vi "fligh_simulator.vi"() -> ()   [LabVIEW 2017]
uses:
  <vilib>/Utility/miscctls.llb/LV3DPointTypeDef.ctl
  nmea/NMEA_GPVTG-data.ctl
  nmea/NMEA_Mode.ctl
  nmea/NMEA_GPRMC-data.ctl
  nmea/NMEA_LatitudeDirection.ctl
  nmea/NMEA_LongitudeDirection.ctl
  nmea/NMEA_GPGGA-data.ctl
  nmea/NMEA_GPS-Quality.ctl
  Program Files (x86)/National Instruments/LabVIEW 2017/examples/Instrument IO/Serial/support/Serial - Settings.ctl
  Program Files (x86)/National Instruments/LabVIEW 2017/examples/Instrument IO/Serial/support/Serial - XON-XOFF Characters.ctl
  Program Files (x86)/National Instruments/LabVIEW 2017/examples/Instrument IO/Serial/support/Serial - ASCII Characters.ctl
  <vilib>/Instr/_visa.llb/VISA Flush IO Buffer Mask.ctl
  Simflight/Attachments from Google Maps in LabVIEW/Attachments from Google Maps in LabVIEW/Google Maps_LV2012_NI Verified/Google Maps_LV2012_NI Verified/SubVIs/States.ctl
  Program Files (x86)/National Instruments/LabVIEW 2017/examples/Connectivity/Web Services/Weather Monitor/Application/Weather Data.ctl
  <vilib>/Instr/_visa.llb/VISA Configure Serial Port (Instr).vi
  Attitude Indicator 2012 NIVerified/Attitude Indicator 2012 NIVerified/lv-attitudecontrol.lvlib
  Downloads/NMEA_v1.1.2 LV2014/NMEA_v1.1/NMEA.lvlib
  Program Files (x86)/National Instruments/LabVIEW 2017/examples/Connectivity/Web Services/Weather Monitor/Application/Weather Data.lvlib
panel:
  in  "sagsol":dbl(slide) scale=-128.0..128.0
  in  "yukarý":dbl(slide) scale=-128.0..128.0
  out "Waveform Graph":dbl[](graph)
  out "Numeric":dbl format="%#_5g"
  in  "Stop 4":bool
  out "Temperature":dbl
  out "Pressure":dbl
  out "Wind Speed":dbl
  out "Wind Direction":dbl
  in  "Update interval":i32=1000
  in  "Slicon L.":refnum<visa-resource-name>="COM1"
  in  "PROLIFIC":refnum<visa-resource-name>
  out "?":dbl format="%#_4g"
  out "GPS Connection":bool
  in  "WebBrowser":refnum<k7>(container)
  in  "Path Color":u32(colorbox)=16729106
  in  "Weight":i32=7
  in  "Location 1":string(combo)="A"
  in  "Location 2":string(combo)="B"
  in  "Latitude":dbl=51.4062 format="%#.6g"
  in  "Longitude":dbl=-1.3070000000000026 format="%#.6g"
  in  "Zoom":sgl=16.0 format="%#.1g"
  in  "Size Y":dbl=650.0
  in  "Size X":dbl=450.0
  in  "Map Format":string(combo)="roadmap"
  in  "Stop 3":bool
  in  "Add Marker?":bool
  in  "Show Path?":bool
  in  "Refresh Button":bool
  out "Gravity":dbl
  out "Acceleration Y":dbl(slide) scale=-1000.0..1000.0
  out "Acceleration X":dbl(slide) scale=-1000.0..1000.0
  out "ivme z":string
  out "ivme y":string
  out "ivme x":string
  out "Gyro Z":dbl(slide) scale=-1000.0..1000.0
  out "Gyro Y":dbl(slide) scale=-90.0..90.0
  out "Gyro X":dbl(slide) scale=-90.0..90.0
  out "gyro y":string
  out "gyro x":string
  out "Speed in km/h":dbl
  out "PRESSURE\n(ATM)":dbl(knob) scale=0.9..1.2
  out "XY Graph 3":cluster{dbl[], dbl[]}(graph)={[1.6583], [1.60678]}
  out "XY Graph 2":cluster{dbl[], dbl[]}(graph)={[1.6583], [1.60678]}
  out "Battery":dbl(slide) scale=0.1..100.0
  out "Battery":bool
  out "Communication":bool
  out "Temperature":bool
  out "Altitude":bool
  out "Flight Mode":string
  out "Flying":bool
  out "GPS-Quality":T1
  out "Universal\nTime\nCoordinated":timestamp format="%<%I:%M:%S>T"
  out "Altitude":dbl(slide) scale=0.0..500.0
  out "Number of Satellites":i32
  out "Temperature":dbl(slide) scale=0.0..100.0
  out "Speed in Knots":dbl(knob) scale=0.0..10.0
  out "Rx":dbl
  out "Temperature":dbl
  out "Ry":dbl
  out "BASINÇ ATM":dbl
  out "gyro z":string
  out "ry":string
  out "rx":string
  out "BASINÇ":string
  out "Temperature":string
  in  "Termination Character":u8=10 format="%.0x"
  in  "End Write on Termination Character?":bool=TRUE
  in  "XON/XOFF Characters":T2={"XON"=enum."DC1", "XOFF"=enum."DC3"}
  in  "Serial Settings":T4={"baud rate"=9600, "data bits"=8, "parity"=enum."None", "stop bits"=10, "flow control"=0} {"flow control" items=["None"=0, "XON/XOFF"=1, "RTS/CTS"=2, "DTR/DSR"=4]; "stop bits" items=["1.0"=10, "1.5"=15, "2.0"=20]; "data bits" min=5 max=8 step=1; "baud rate" items=["75"=75, "110"=110, "134"=134, "150"=150, "300"=300, "600"=600, "1200"=1200, "1800"=1800, "2400"=2400, "4800"=4800, "7200"=7200, "9600"=9600, "14400"=14400, "19200"=19200, "28800"=28800, "38400"=38400, "56000"=56000, "57600"=57600, "115200"=115200, "128000"=128000, "230400"=230400]}
  in  "End Read on Termination Character?":bool=TRUE
  out "Response":string
  in  "Read Count":u32=1000
  in  "connect":bool
  in  "Stop 2":bool
  in  "Buffer Size":u32=6400
  out "$GPGGA-message_OUT":T5={"TimeStamp"=timestamp(0 s since 1904-01-01), "Latitude"=0.0, "Latitude-Direction"=enum."", "Longitude"=1.0, "Longitude-Direction"=enum."", "GPS-Quality"=enum."GPS fix (SPS)", "Number of Satellites"=0, "Horizontal Dilution of Precision"=0.0, "Altitude above Mean-Sea-Level"=0.0, "Geoidal separation"=0.0, "Time since last DGPS update"=0.0, "DGPS reference station ID"=0} {"Time since last DGPS update" format="%.02f [s]"; "Geoidal separation" format="%.02f [m]"; "Altitude above Mean-Sea-Level" format="%.02f [m]"; "Horizontal Dilution of Precision" format="%.02f [HDOP]"; "Longitude" format="%0.4f [long]"; "Latitude" format="%.04f [lat]"; "TimeStamp" format="%<%.2X>T"}
  out "LATITUDE":dbl
  out "LONGITUDE":dbl
  out "Data":string[][](table)
  out "$GPRMC-message_OUT":T8={"TimeStamp"=timestamp(0 s since 1904-01-01), "Validity"=FALSE, "Latitude"=0.0, "Latitude-Direction"=enum."North", "Longitude"=0.0, "Longitude-Direction"=enum."East", "Speed in knots"=0.0, "True course"=0.0, "Date Stamp"=timestamp(0 s since 1904-01-01), "Magnetic Variation (East/West)"=0.0} {"Magnetic Variation (East/West)" format="%.02f [deg]"; "Date Stamp" format="%<%x>T"; "True course" format="%.02f [deg]"; "Speed in knots" format="%.02f [kts]"; "Longitude" format="%0.4f [long]"; "Latitude" format="%.04f [lat]"; "TimeStamp" format="%<%.2X>T"}
  out "$GPVTG-message_OUT":T9={"True Course over Ground"=0.0, "Magnetic Course over Ground"=0.0, "Speed over Ground in knots"=0.0, "Speed over Ground in km/h"=1.0, "Mode"=""} {"Speed over Ground in km/h" format="%.02f [km/h]"; "Speed over Ground in knots" format="%.02f [kts]"; "Magnetic Course over Ground" format="%.02f [deg]"; "True Course over Ground" format="%.02f [deg]"}
  out "NMEA":string
  in  "Stop":bool
  in  "Control 1":T11 {"X" scale=-90.0..90.0; "Y" scale=-180.0..180.0; "Z" scale=0.0..360.0}
  in  "stop":bool
  in  "pusula":dbl(slide) max=360.0 scale=0.0..360.0
  in  "pusula stop":bool
  out "Gauge":dbl(knob) scale=0.0..360.0
  in  "Attitude Indicator":refnum<vi>(3d-picture)
  # "Flight Status"
  # "UTC"
  # "NOTIFICATIONS"
  # "STATION"
  # "SELCUK ALTINAY\nHAKAN GURBUZ"
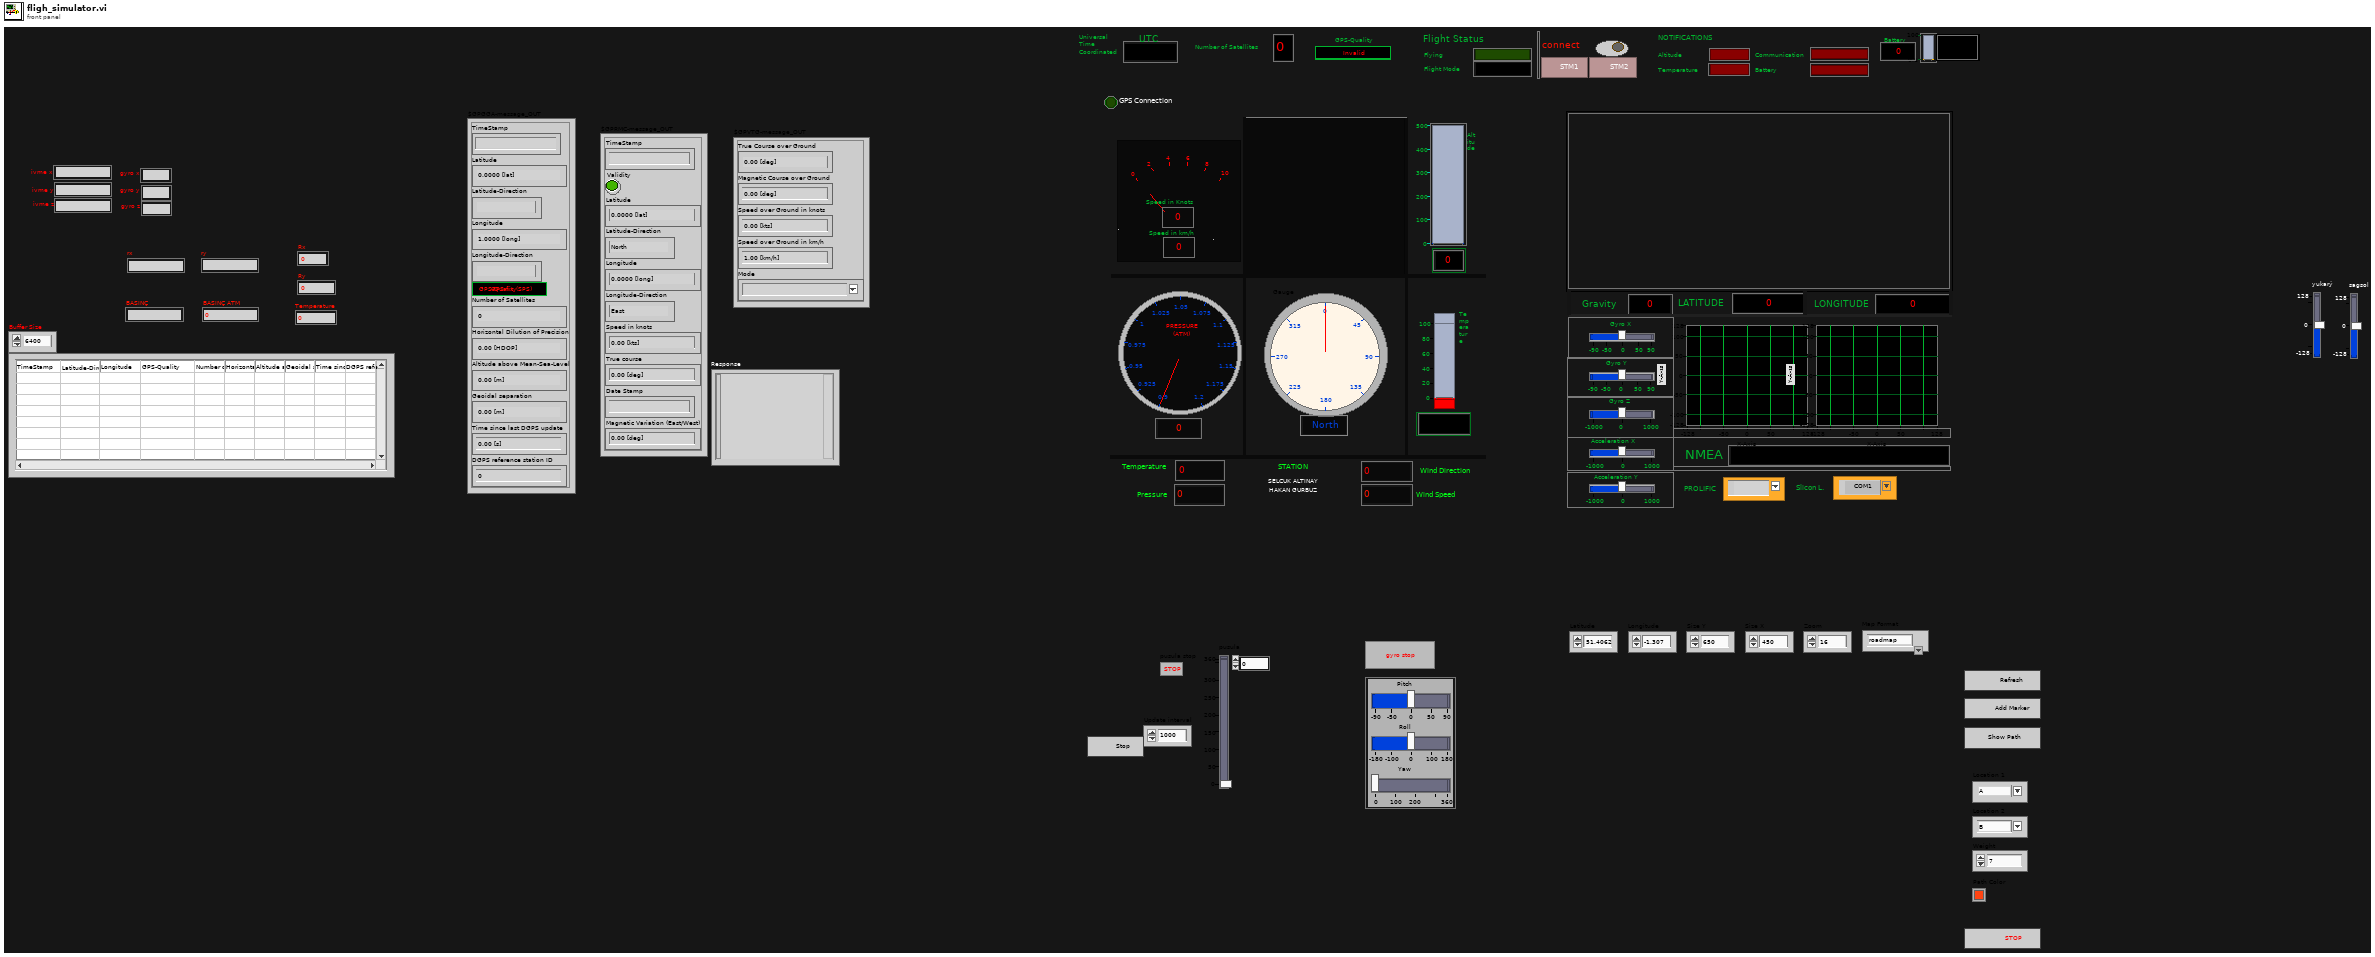
[diagram p1: front panel]
types:
  T1 = typedef "NMEA.lvlib/NMEA_GPS-Quality.ctl" = enum16{"Invalid", "GPS fix (SPS)", "DGPS fix", "PPS fix", "Real Time Kinematic", "Float RTK", "estimated", "Manual input mode", "Simulation mode"}
  T2 = typedef "Serial - XON-XOFF Characters.ctl" = cluster{"XON":T3, "XOFF":T3}
  T3 = typedef "Serial - ASCII Characters.ctl" = enum16{"NUL", "SOH", "STX", "ETX", "EOT", "ENQ", "ACK", "BEL", "BS", "HT", "LF", "VT", "FF", "CR", "SO", "SI", "DLE", "DC1", "DC2", "DC3", "DC4", "NAK", "SYN", "ETB", "CAN", "EM", "SUB", "ESC", "FS", "GS", "RS", "US", "SP", "!", "\"", "#", "$", "%", "&", "'", "(", ")", "*", "+", ",", "- (-)", ".", "/", "0", "1", "2", "3", "4", "5", "6", "7", "8", "9", ":", ";", "<", "=", ">", "?", "@", "A", "B", "C", "D", "E", "F", "G", "H", "I", "J", "K", "L", "M", "N", "O", "P", "Q", "R", "S", "T", "U", "V", "W", "X", "Y", "Z", "[", "\\", "]", "^", "_", "`", "a", "b", "c", "d", "e", "f", "g", "h", "i", "j", "k", "l", "m", "n", "o", "p", "q", "r", "s", "t", "u", "v", "w", "x", "y", "z", "{", "|", "}", "~"}
  T4 = typedef "Serial - Settings.ctl" = cluster{"baud rate":u32, "data bits":u16, "parity":enum16{"None", "Odd", "Even", "Mark", "Space"}, "stop bits":u16, "flow control":u16}
  T5 = typedef "NMEA.lvlib/NMEA_GPGGA-data.ctl" = cluster{"TimeStamp":timestamp, "Latitude":dbl, "Latitude-Direction":T6, "Longitude":dbl, "Longitude-Direction":T7, "GPS-Quality":T1, "Number of Satellites":i32, "Horizontal Dilution of Precision":dbl, "Altitude above Mean-Sea-Level":dbl, "Geoidal separation":dbl, "Time since last DGPS update":dbl, "DGPS reference station ID":i32}
  T6 = typedef "NMEA.lvlib/NMEA_LatitudeDirection.ctl" = enum16{"", "North", "South"}
  T7 = typedef "NMEA.lvlib/NMEA_LongitudeDirection.ctl" = enum16{"", "East", "West"}
  T8 = typedef "NMEA.lvlib/NMEA_GPRMC-data.ctl" = cluster{"TimeStamp":timestamp, "Validity":bool, "Latitude":dbl, "Latitude-Direction":T6, "Longitude":dbl, "Longitude-Direction":T7, "Speed in knots":dbl, "True course":dbl, "Date Stamp":timestamp, "Magnetic Variation (East/West)":dbl}
  T9 = typedef "NMEA.lvlib/NMEA_GPVTG-data.ctl" = cluster{"True Course over Ground":dbl, "Magnetic Course over Ground":dbl, "Speed over Ground in knots":dbl, "Speed over Ground in km/h":dbl, "Mode":T10}
  T10 = typedef "NMEA.lvlib/NMEA_Mode.ctl" = string
  T11 = typedef "LV3DPointTypeDef.ctl" = cluster{"X":sgl, "Y":sgl, "Z":sgl}
  T12 = cluster{"Marker":string, "Path":string, "Markers Coordinates":string[][]}
  T13 = typedef "States.ctl" = enum16{"Wait on Event", "Update Map", "Add Marker", "Show Path", "Shutdown"}
  T14 = typedef "VISA Flush IO Buffer Mask.ctl" = u16
  T15 = typedef "Weather Data.lvlib/Weather Data.ctl" = cluster{"Temperature":dbl, "Pressure":dbl, "Wind Speed":dbl, "Wind Direction":dbl}
  T16 = typedef "lv-attitudecontrol.lvlib/AttitudeHandle.ctl" = cluster{"First Scene Object":refnum<vi>, "Drum":refnum<vi>, "Window":refnum<vi>, "Dial":refnum<vi>, "Scene Graph":refnum<vi>, "Last Drum Pitch":dbl, "Last Drum Roll ":dbl, "Last Dial Roll":dbl}
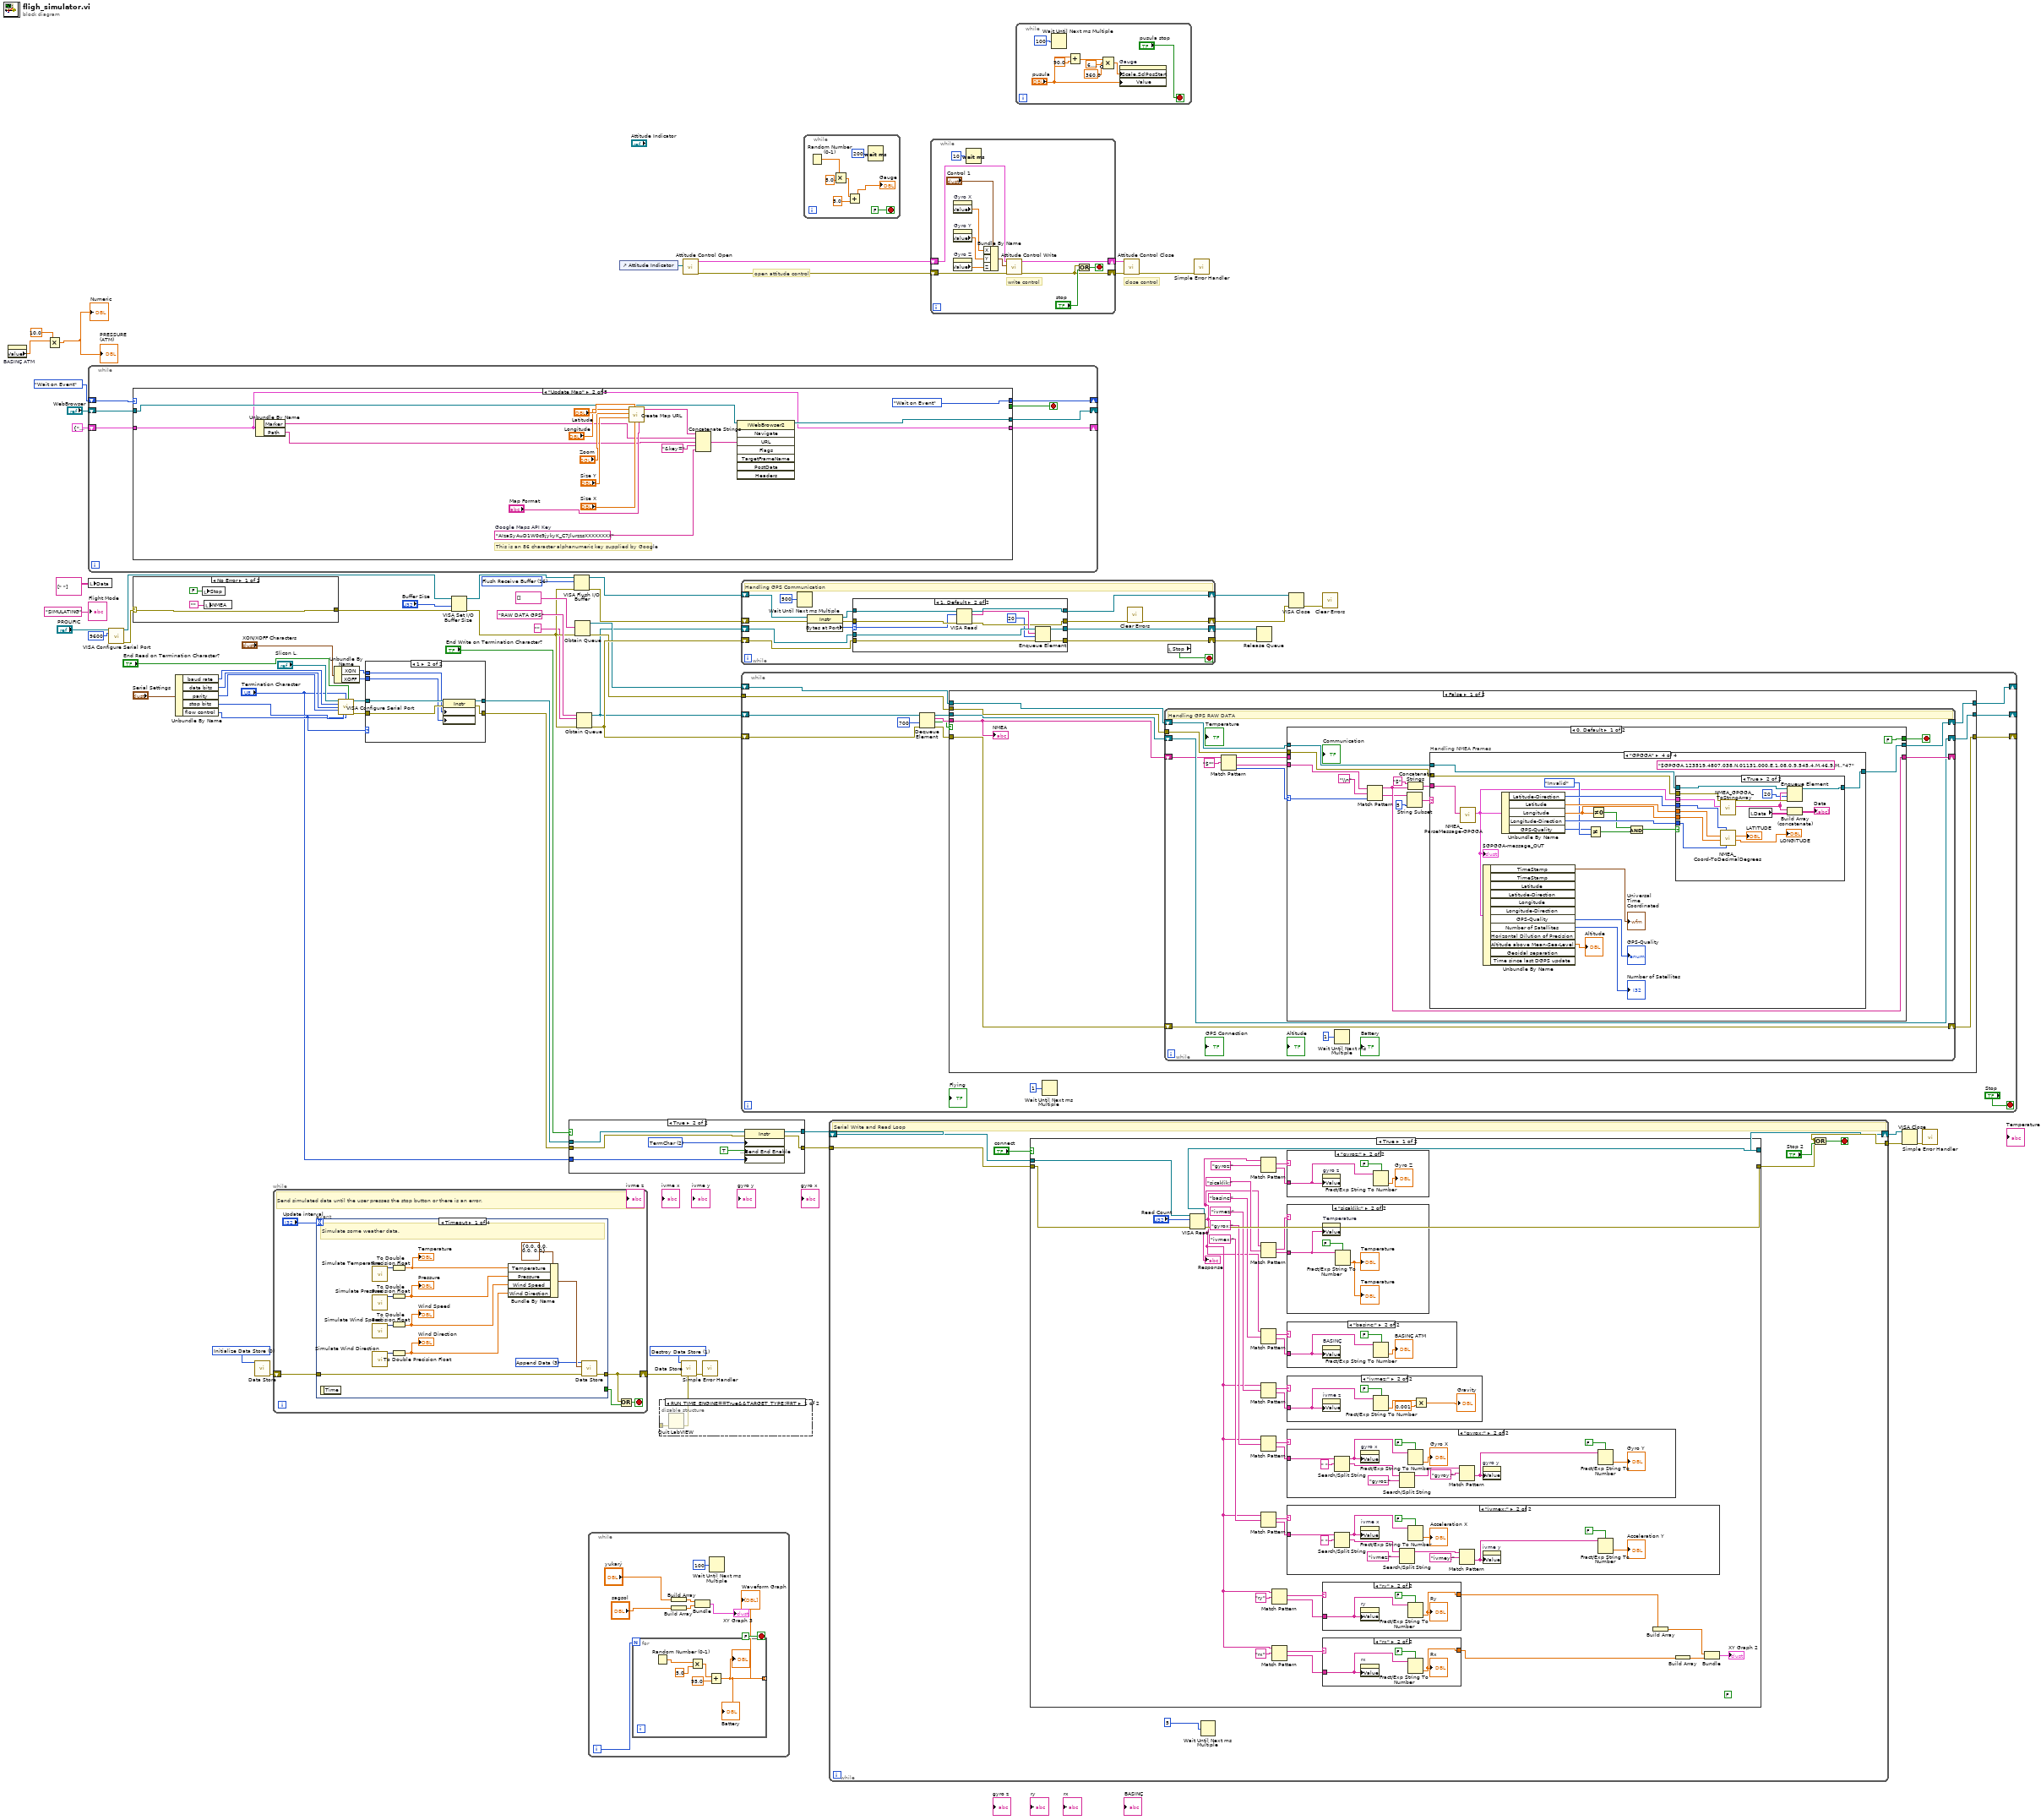
[diagram p0: block diagram]
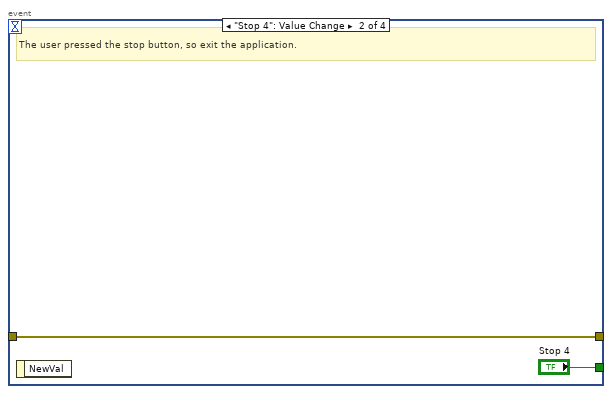
[diagram p3: hidden frame]
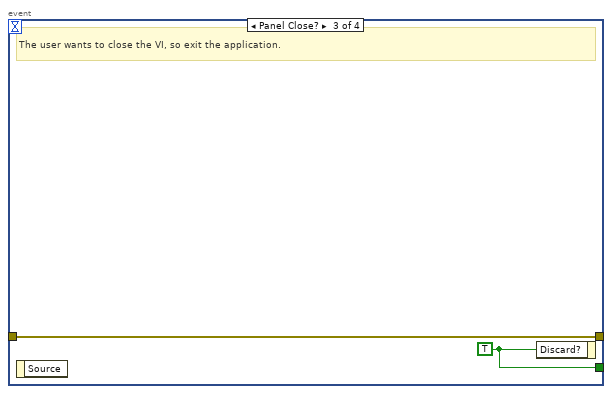
[diagram p4: hidden frame]
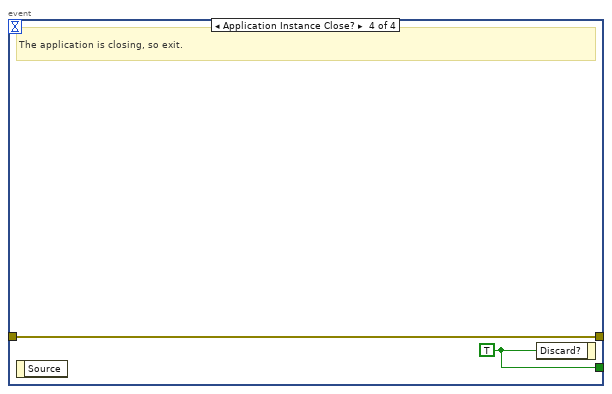
[diagram p5: hidden frame]
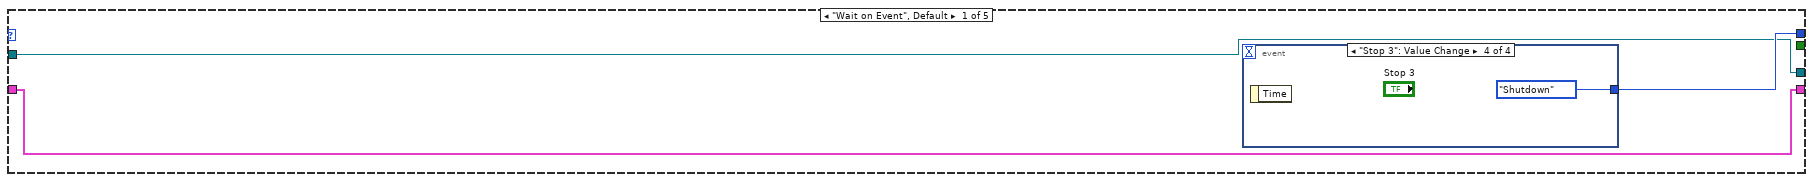
[diagram p6: hidden frame]
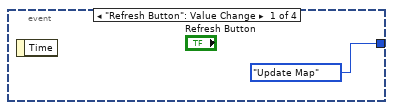
[diagram p7: hidden frame]
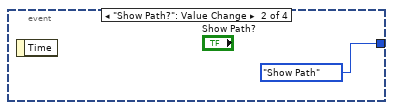
[diagram p8: hidden frame]
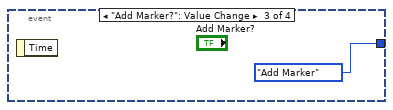
[diagram p9: hidden frame]
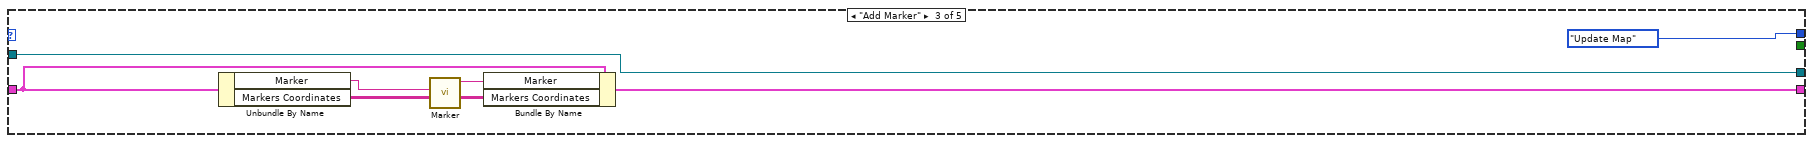
[diagram p10: hidden frame]
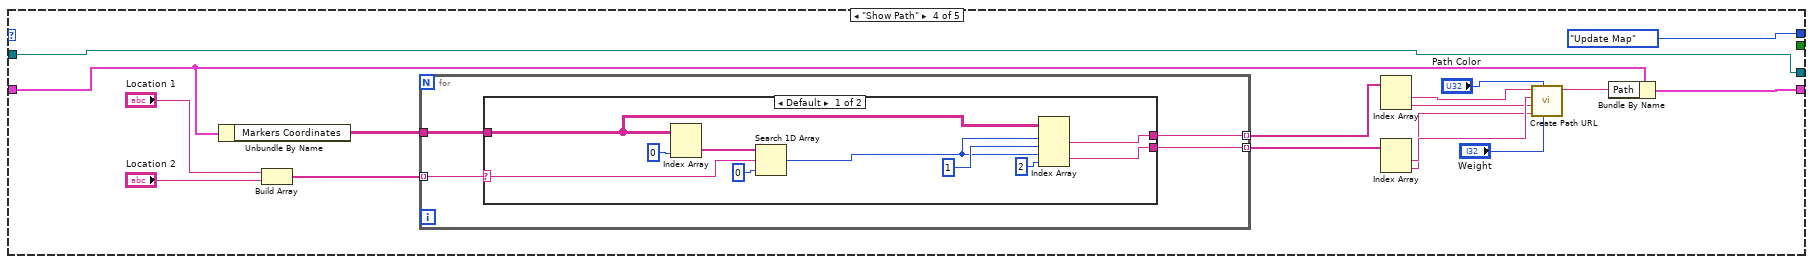
[diagram p11: hidden frame]
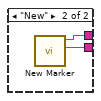
[diagram p12: hidden frame]
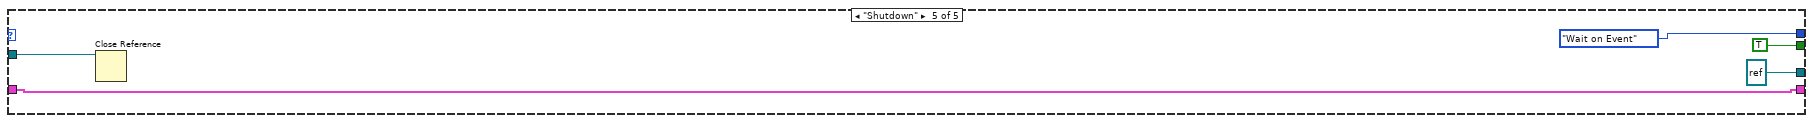
[diagram p13: hidden frame]
diagram:
  w8 = u16 1 items=["Initialize Data Store", "Destroy Data Store", "Clear Data", "Append Data", "Get Last Data", "Get All Data"] ("action")
  w5 = u16 0 items=["Initialize Data Store", "Destroy Data Store", "Clear Data", "Append Data", "Get Last Data", "Get All Data"] ("action")
  w49 = T14 16 items=["Flush Receive Buffer"=16, "Write Transmit Buffer to Device"=32, "Flush Receive Buffer (No I/O)"=64, "Flush Transmit Buffer"=128] ("Mask")
  # "close control"
  # "open attitude control"
  n1 = property on="BASINÇ ATM" class="DigNum (strict)"() -> ("Value"=w3:dbl)  [unwired: 2 in, 2 out]
  n2 = Multiply(x=w3, y=10.0) -> (x*y=→"PRESSURE\n(ATM)" →"Numeric":dbl)
  n3 = while {
    shift-right: [w72] -> _
    shift-left: States."Wait on Event" -> [w71]
    shift-right: [w69] -> _
    shift-left: "WebBrowser" -> [w68]
    shift-right: [w66] -> _
    shift-left: T12 {"Marker"="", "Path"="", "Markers Coordinates"=[]} -> [w67]
    stop <- w70 stop-if-true
    n4 = case shown="\"Update Map\"" w71 {
      tunnel: [w75 States."Wait on Event" States."Update Map" States."Update Map" States."Wait on Event"] -> w72
      tunnel: [_ _ _ _ TRUE] -> w70
      tunnel: w68 -> [w74 w87 w103 w120 w140]
      tunnel: [w74 w86 w103 w120 refnum<k7> refnum ("WebBrowser")] -> w69
      tunnel: w67 -> [w73 w80 w99 w109 w137]
      tunnel: [w73 w80 w96 w108 w137] -> w66
      frame "Wait on Event", Default {
        n5 = event shown="[3] \"Stop 3\": Value Change" {
          selector: _ -> [_ _ _ _]
          dyn-events: _ -> [_ _ _ _]
          timeout: _ -> [_ _ _ _]
          tunnel: [States."Update Map" States."Show Path" States."Add Marker" States."Shutdown"] -> w75
          event "Refresh Button": Value Change {
            n6 = event-data() -> ()  [unwired: 1 in, 1 out]
          }
          event "Show Path?": Value Change {
            n7 = event-data() -> ()  [unwired: 1 in, 1 out]
          }
          event "Add Marker?": Value Change {
            n8 = event-data() -> ()  [unwired: 1 in, 1 out]
          }
          event "Stop 3": Value Change {
            n9 = event-data() -> ()  [unwired: 1 in, 1 out]
          }
        }
      }
      frame "Update Map" {
        w83 = "AIzaSyAuD1W0c9jykyK_C7JlurzzsXXXXXXXX"  # Google Maps API Key
        # "This is an 86 character alphanumeric key supplied by Google"
        n10 = Unbundle By Name(w80) -> ("Marker"=w82:string, "Path"=w81:string)
        n11 = call "Create Map URL.vi"("Map Format"="Map Format", "X"="Size X", "Lat"="Latitude", "Y"="Size Y", "Zoom"="Zoom", "Lon"="Longitude") -> ("String"=w89:string)  [unwired: 5 in]
        n12 = Concatenate Strings(w89, w82, w81, "&key=" ("string"), w83) -> (w88:string)
        n13 = invoke class="IWebBrowser2" method="Navigate"(reference=w87, "URL"=w88) -> (reference out=w86:refnum<k7>)  [unwired: 6 in, 7 out]
      }
      frame "Add Marker" {
        n14 = Unbundle By Name(w99) -> ("Marker"=w101:string, "Markers Coordinates"=w100:string[][])
        n15 = call "Marker.vi"("Markers in"=w100, "Initial String"=w101) -> ("Markers out"=w97:string[][], "Balloon"=w98:string)  [unwired: 8 in]
        n16 = Bundle By Name(cluster=w99, "Marker"=w98, "Markers Coordinates"=w97) -> (w96:T12)
      }
      frame "Show Path" {
        n17 = Unbundle By Name(w109) -> ("Markers Coordinates"=w111:string[][])
        n18 = Build Array("Location 1", "Location 2") -> (w116:string[])
        n19 = for {
          tunnel: w116 -> [w124] mode=indexing
          tunnel: [w123] -> w115 mode=indexing
          tunnel: [w122] -> w114 mode=indexing
          tunnel: w111 -> [w121]
          n20 = case shown="Default" w124 {
            selector: w124 -> [w125 _]
            tunnel: [w127 w136] -> w123
            tunnel: [w126 w135] -> w122
            tunnel: w121 -> [w128 _]
            frame Default {
              n21 = Index Array(array=w128, index (col)=0 ("disabled index (col)")) -> (element=w129:string[])  [unwired: 1 in]
              n22 = Search 1D Array(1D array=w129, element=w125, start index (0)=0) -> (index of element=w132:i32)
              n23 = Index Array(array=w128, index (row) #1=w132, index (col) #1=1 ("disabled index (col)"), index (row) #2=w132, index (col) #2=2 ("disabled index (col)")) -> (element #1=w127:string, element #2=w126:string)
            }
            frame "New" {
              n24 = call "New Marker.vi"() -> ("Longitude"=w135:string, "Latitude"=w136:string)  [unwired: 10 in]
            }
          }
        }
        n25 = Index Array(array=w115) -> (element #1=w112:string, element #2=w105:string)  [unwired: 2 in]
        n26 = Index Array(array=w114) -> (element #1=w106:string, element #2=w104:string)  [unwired: 2 in]
        n27 = call "Create Path URL.vi"("Weight"="Weight", "Path Collor"="Path Color", "Long Point 2"=w104, "Lat Point 2"=w105, "Long Point 1"=w106, "Lat Point 1"=w112) -> ("String 4"=w110:string)  [unwired: 5 in]
        n28 = Bundle By Name(cluster=w109, "Path"=w110) -> (w108:T12)
      }
      frame "Shutdown" {
        n29 = Close Reference(reference=w140) -> ()  [unwired: 1 in, 1 out]
      }
    }
  }
  n30 = local write "Data"(string[][] [[" "]]) -> ()
  n31 = call-poly "VISA Configure Serial Port"("VISA resource name"="PROLIFIC", "baud rate (9600)"=u32 9600) -> ("VISA resource name out"=w50:refnum<visa-resource-name>, "error out"=w41:errorcluster)  [unwired: 12 in]
  n32 = case shown="No Error" w41 {
    selector: w41 -> [w143 w145]
    tunnel: [w143 w145] -> w39
    frame No Error {
      n33 = local write "Stop"(FALSE ("STOP")) -> ()
      n34 = local write "NMEA"("") -> ()
    }
    frame Error {
    }
  }
  n35 = Unbundle By Name("Serial Settings") -> ("baud rate"=w28:u32, "data bits"=w29:u16, "parity"=w30:enum16{"None", "Odd", "Even", "Mark", "Space"}, "stop bits"=w31:u16, "flow control"=w22:u16)
  n36 = call "Data Store.vi"("action"=w5) -> ("error out"=w6:errorcluster)  [unwired: 9 in, 1 out]
  n37 = while {
    shift-right: [w148] -> w7
    shift-left: w6 -> [w150]
    stop <- w149 stop-if-true
    # "Send simulated data until the user presses the stop button or there is an error."
    n38 = event shown="[0] Timeout" {
      selector: _ -> [_ _ _ _]
      dyn-events: _ -> [_ _ _ _]
      timeout: "Update interval" -> [_ _ _ _]
      tunnel: w150 -> [w159 w165 w167 w169]
      tunnel: [w157 w165 w167 w169] -> w148
      tunnel: [_ "Stop 4" w166 w168] -> w146
      event Timeout {
        w151 = u16 3 items=["Initialize Data Store", "Destroy Data Store", "Clear Data", "Append Data", "Get Last Data", "Get All Data"] ("action")
        # "Simulate some weather data."
        n39 = event-data() -> ()  [unwired: 1 in, 1 out]
        n40 = call "Simulate Temperature"() -> ("DC with Uniform Noise"=w156:dynamicdata)  [unwired: 5 in, 10 out]
        n41 = call "Simulate Pressure"() -> ("Sine with Uniform Noise"=w162:dynamicdata)  [unwired: 8 in, 7 out]
        n42 = call "Simulate Wind Speed"() -> ("Sine with Uniform Noise"=w161:dynamicdata)  [unwired: 8 in, 7 out]
        n43 = call "Simulate Wind Direction"() -> ("Sine with Uniform Noise"=w160:dynamicdata)  [unwired: 8 in, 7 out]
        n44 = To Double Precision Float(number=w156) -> (double precision float=w155:dbl)
        "Temperature" <- w155
        n45 = To Double Precision Float(number=w162) -> (double precision float=w154:dbl)
        "Pressure" <- w154
        n46 = To Double Precision Float(number=w161) -> (double precision float=w153:dbl)
        "Wind Speed" <- w153
        n47 = To Double Precision Float(number=w160) -> (double precision float=w152:dbl)
        "Wind Direction" <- w152
        n48 = Bundle By Name(cluster=T15 {"Temperature"=0.0, "Pressure"=0.0, "Wind Speed"=0.0, "Wind Direction"=0.0} ("Weather Data"), "Temperature"=w155, "Pressure"=w154, "Wind Speed"=w153, "Wind Direction"=w152) -> (w158:T15)
        n49 = call "Data Store.vi"("error in (no error)"=w159, "new weather data"=w158, "action"=w151) -> ("error out"=w157:errorcluster)  [unwired: 7 in, 1 out]
      }
      event "Stop 4": Value Change {
        # "The user pressed the stop button, so exit the application."
        n50 = event-data() -> ()  [unwired: 1 in, 1 out]
      }
      event Panel Close? {
        w166 = TRUE ("Discard?")
        # "The user wants to close the VI, so exit the application."
        n51 = event-data() -> ()  [unwired: 1 in, 1 out]
        n52 = event-data("Discard?"=w166) -> ()  [unwired: 1 in, 1 out]
      }
      event Application Instance Close? {
        w168 = TRUE ("Discard?")
        # "The application is closing, so exit."
        n53 = event-data() -> ()  [unwired: 1 in, 1 out]
        n54 = event-data("Discard?"=w168) -> ()  [unwired: 1 in, 1 out]
      }
    }
    n55 = Or(x=w148, y=w146) -> (x .or. y?=w149:bool)
  }
  n56 = Unbundle By Name("XON/XOFF Characters") -> ("XON"=w21:T3, "XOFF"=w20:T3)
  n57 = call-poly "VISA Configure Serial Port"("VISA resource name"="Slicon L.", "termination char\n(0xA = '\\n' = LF)"="Termination Character", "Enable Termination\nChar (T)"="End Read on Termination Character?", "baud rate (9600)"=w28, "data bits (8)"=w29, "parity (0:none)"=w30, "stop bits (10: 1 bit)"=w31, "flow control (0:none)"=w22) -> ("VISA resource name out"=w32:refnum<visa-resource-name>, "error out"=w33:errorcluster)  [unwired: 2 in, 4 out]
  n58 = case shown="1" w22 {
    tunnel: [w170 w177] -> w19
    tunnel: [w171 w176] -> w17
    tunnel: w33 -> [w170 w175]
    tunnel: w32 -> [w171 w174]
    tunnel: w21 -> [_ w173]
    tunnel: w20 -> [_ w172]
    frame Default {
    }
    frame 1 {
      n59 = property class="Instr"(reference=w174, error in=w175, "Serial Settings:Flow Control XON Character"=w173, "Serial Settings:Flow Control XOFF Character"=w172) -> (reference out=w176:refnum<visa-resource-name>, error out=w177:errorcluster)
    }
  }
  n60 = VISA Set I/O Buffer Size(VISA resource name=w50, size (4096)="Buffer Size", error in (no error)=w39) -> (VISA resource name out=w59:refnum<visa-resource-name>, error out=w38:errorcluster)  [unwired: 1 in]
  n61 = case shown="True" "End Write on Termination Character?" {
    tunnel: w17 -> [w178 w186]
    tunnel: w19 -> [w179 w185]
    tunnel: [w178 w184] -> w16
    tunnel: [w179 w183] -> w18
    tunnel: "Termination Character" -> [_ w181]
    frame False {
    }
    frame True {
      w182 = u16 2 items=["None", "LastBit", "TermChar", "Break"] ("Serial Settings:Serial End Mode for Writes")
      n62 = property class="Instr"(reference=w186, error in=w185, "Serial Settings:End Mode for Writes"=w182, "Message Based Settings:Send End Enable"=TRUE, "Message Based Settings:Termination Character"=w181) -> (reference out=w184:refnum<visa-resource-name>, error out=w183:errorcluster)
    }
  }
  n63 = VISA Flush I/O Buffer(VISA resource name=w59, mask (16)=w49, error in (no error)=w38) -> (VISA resource name out=w58:refnum<visa-resource-name>, error out=w57:errorcluster)
  n64 = Obtain Queue(element data type=string[] [], error in (no error)=w38) -> (queue out=w55:refnum<queue>, error out=w54:errorcluster)  [unwired: 3 in, 1 out]
  n65 = Obtain Queue(name (unnamed)="RAW DATA GPS" ("nom (aucun)"), element data type="" ("expression régulière"), error in (no error)=w38) -> (queue out=w45:refnum<queue>, error out=w56:errorcluster)  [unwired: 2 in, 1 out]
  n66 = while {
    i -> [w187]
    stop <- FALSE stop-if-true
    n67 = for {
      N: w187 -> [_]
      tunnel: [w196] -> w188 mode=indexing
      n68 = Random Number (0-1)() -> (number: 0 to 1=w200:dbl)
      n69 = Multiply(x=w200, y=5.0) -> (x*y=w198:dbl)
      n70 = Add(x=w198, y=95.0) -> (x+y=w196:dbl)
      "Battery" <- w196
      "?" <- w196
    }
    "Waveform Graph" <- w188
    n71 = Build Array("yukarý") -> (w195:dbl[])
    n72 = Build Array("sagsol") -> (w194:dbl[])
    n73 = Bundle(w195, w194) -> (→"XY Graph 3":cluster{dbl[], dbl[]})  [unwired: 1 in]
    n74 = Wait Until Next ms Multiple(millisecond multiple=u32 100) -> ()  [unwired: 1 out]
  }
  n75 = control-ref of="Attitude Indicator"() -> (w62:refnum<vi>)
  n76 = call "Data Store.vi"("error in (no error)"=w7, "action"=w8) -> ("error out"=w4:errorcluster)  [unwired: 8 in, 1 out]
  n77 = call "Attitude Control Open.vi"("Scene Graph"=w62) -> ("error out"=w61:errorcluster, "Attitude Control Handle"=w60:T16)  [unwired: 9 in]
  n78 = call <vilib>:"Simple Error Handler.vi"("error in (no error)"=w4) -> ("error out"=w9:errorcluster)  [unwired: 4 in, 4 out]
  n79 = disable-structure shown="RUN_TIME_ENGINE==True&&TARGET_TYPE!=RT" {
    disable-tunnel: w9 -> [_ _]
    frame condition #0 {
      n80 = Quit LabVIEW() -> ()  [unwired: 1 in]
    }
    frame condition #1 (active) {
    }
  }
  n81 = while {
    shift-right: [w211] -> w47
    shift-left: w56 -> [w213]
    shift-right: [w210] -> w44
    shift-left: w58 -> [w209]
    shift-right: [w212] -> w46
    shift-left: w45 -> [w214]
    shift-right: [w202] -> w43
    shift-left: w57 -> [w206]
    stop <- w201 stop-if-true
    # "Handling GPS Communication"
    n82 = Wait Until Next ms Multiple(millisecond multiple=u32 500 ("attente (ms)")) -> ()  [unwired: 1 out]
    n83 = property class="Instr"(reference=w209, error in=w206) -> (reference out=w208:refnum<visa-resource-name>, error out=w205:errorcluster, "Bytes at Port"=w203:u32)
    n84 = case shown="1, Default" w203 {
      selector: w203 -> [_ w220]
      tunnel: w214 -> [w215 w229]
      tunnel: w213 -> [w216 w228]
      tunnel: [w215 w227] -> w212
      tunnel: [w216 w226] -> w211
      tunnel: [w217 w224] -> w210
      tunnel: w208 -> [w217 w223]
      tunnel: w205 -> [w218 w222]
      tunnel: [w218 w221] -> w204
      frame 0 {
      }
      frame 1, Default {
        n85 = VISA Read(VISA resource name=w223, byte count=w220, error in (no error)=w222) -> (VISA resource name out=w224:refnum<visa-resource-name>, read buffer=w225:string, error out=w221:errorcluster)  [unwired: 1 out]
        n86 = Enqueue Element(queue=w229, element=w225, timeout in ms (-1)=20 ("timeout en ms (-1)"), error in (no error)=w228) -> (queue out=w227:refnum<queue>, error out=w226:errorcluster)  [unwired: 1 out]
      }
    }
    n87 = call <vilib>:"Clear Errors.vi"("error in (no error)"=w204) -> ("error out"=w202:errorcluster)  [unwired: 5 in, 1 out]
    n88 = local read "Stop"() -> (w201:bool)
  }
  n89 = while {
    tunnel: w54 -> [w239]
    shift-right: [w237] -> _
    shift-left: w45 -> [w238]
    shift-right: [w233] -> _
    shift-left: w55 -> [w240]
    shift-right: [w232] -> _
    shift-left: w56 -> [w243]
    stop <- "Stop" stop-if-true
    n90 = Dequeue Element(queue=w238, timeout in ms (-1)=700 ("timeout en ms (-1)"), error in (no error)=w243) -> (queue out=w236:refnum<queue>, element=w242:string, timed out?=w234:bool, error out=w231:errorcluster)
    n91 = case shown="False" w234 {
      tunnel: w242 -> [w244 _]
      tunnel: w240 -> [w251 w324]
      tunnel: w239 -> [w250 _]
      tunnel: [w249 w325] -> w237
      tunnel: w236 -> [w248 w325]
      tunnel: [w247 w324] -> w233
      tunnel: [w246 w323] -> w232
      tunnel: w231 -> [w245 w323]
      frame False {
        n92 = while {
          shift-right: [w262] -> _
          shift-left: w244 -> [w253]
          tunnel: w250 -> [w258]
          shift-right: [w257] -> w249
          shift-left: w248 -> [w257]
          shift-right: [w255] -> w247
          shift-left: w251 -> [w259]
          shift-right: [w254] -> w246
          shift-left: w245 -> [w254]
          stop <- w256 stop-if-true
          # "Handling GPS RAW DATA"
          n93 = Match Pattern(string=w253, regular expression="$*" ("expression régulière")) -> (before substring=w252:string, after substring=w261:string, offset past match=w263:i32)  [unwired: 1 in, 1 out]
          n94 = case shown="0, Default" w263 {
            selector: w263 -> [w274 _]
            tunnel: [w273 w320] -> w262
            tunnel: w261 -> [w275 _]
            tunnel: [FALSE TRUE] -> w256
            tunnel: w259 -> [w268 w321]
            tunnel: w258 -> [w267 _]
            tunnel: [w265 w321] -> w255
            tunnel: w252 -> [_ w320]
            frame 0, Default {
              n95 = Match Pattern(string=w275, regular expression="\\n" ("expression régulière"), offset (0)=w274) -> (before substring=w272:string, after substring=w273:string)  [unwired: 2 out]
              n96 = String Subset(string=w272, length (rest)=5 ("longueur (reste)")) -> (substring=w276:string)  [unwired: 1 in]
              n97 = Concatenate Strings("$" ("expression régulière"), w272) -> (w270:string)
              n98 = case "Handling NMEA Frames" shown="\"GPGGA\"" w276 {
                tunnel: w270 -> [_ w282 w286 w304]
                tunnel: w268 -> [w278 w281 w285 w300]
                tunnel: w267 -> [_ _ _ w299]
                tunnel: [w278 w281 w285 w298] -> w265
                frame " ", Default {
                }
                frame "GPVTG" {
                  (unwired) "$GPVTG,054.7,T,034.4,M,005.5,N,010.2,K*48" ("$GPVTG-message_IN")
                  n99 = call "NMEA_ParseMessage-GPVTG.vi"("$GPVTG-message_IN"=w282) -> ("$GPVTG-message_OUT"=w280:T9)  [unwired: 9 in, 1 out]
                  "$GPVTG-message_OUT" <- w280
                  n100 = Unbundle By Name(w280) -> ("Speed over Ground in km/h"=→"Speed in km/h":dbl)  [unwired: 3 out]
                }
                frame "GPRMC" {
                  (unwired) "$GPRMC,225446,A,4916.45,N,12311.12,W,000.5,054.7,191194,020.3,E*68" ("$GPRMC-message_IN")
                  n101 = call "NMEA_ParseMessage-GPRMC.vi"("$GPRMC-message_IN"=w286) -> ("$GPRMC-message_OUT"=w283:T8)  [unwired: 9 in, 1 out]
                  "$GPRMC-message_OUT" <- w283
                  n102 = Unbundle By Name(w283) -> ("Speed in knots"=→"Speed in Knots":dbl)  [unwired: 11 out]
                }
                frame "GPGGA" {
                  (unwired) "$GPGGA,123519,4807.038,N,01131.000,E,1,08,0.9,545.4,M,46.9,M,,*47" ("data out")
                  n103 = call "NMEA_ParseMessage-GPGGA.vi"("$GPGGA-message_IN"=w304) -> ("$GPGGA-message_OUT"=w290:T5)  [unwired: 9 in, 1 out]
                  "$GPGGA-message_OUT" <- w290
                  n104 = Unbundle By Name(w290) -> ("TimeStamp"=→"Universal\nTime\nCoordinated":timestamp, "GPS-Quality"=→"GPS-Quality":T1, "Number of Satellites"=→"Number of Satellites":i32, "Altitude above Mean-Sea-Level"=→"Altitude":dbl)  [unwired: 8 out]
                  n105 = Unbundle By Name(w290) -> ("Latitude-Direction"=w301:T6, "Latitude"=w302:dbl, "Longitude"=w297:dbl, "Longitude-Direction"=w303:T7, "GPS-Quality"=w292:T1)
                  n106 = Not Equal?(x=w292, y=NMEA_GPS-Quality."Invalid" ("GPS-Quality")) -> (x != y?=w293:bool)
                  n107 = Not Equal To 0?(x=w297) -> (x != 0?=w295:bool)
                  n108 = Compound Arithmetic op=AND(w295, w293) -> (w296:bool)
                  n109 = case shown="True" w296 {
                    tunnel: w303 -> [_ w317]
                    tunnel: w302 -> [_ w307]
                    tunnel: w301 -> [_ w306]
                    tunnel: w290 -> [_ w316]
                    tunnel: w300 -> [w305 w315]
                    tunnel: w299 -> [_ w314]
                    tunnel: [w305 w310] -> w298
                    tunnel: w297 -> [_ w308]
                    frame False {
                    }
                    frame True {
                      n110 = call "NMEA_GPGGA_ToStringArray.vi"("$GPGGA-message_IN"=w316) -> ("$GPGGA-message_OUT"=w312:string[])  [unwired: 9 in, 1 out]
                      n111 = call "NMEA_Coord-ToDecimalDegrees.vi"("Longitude-Direction"=w317, "Latitude-Direction"=w306, "Longitude"=w308, "Latitude"=w307) -> ("Longitude"=→"LONGITUDE":dbl, "Latitude"=→"LATITUDE":dbl)  [unwired: 6 in]
                      n112 = local read "Data"() -> (w311:string[][])
                      n113 = Enqueue Element(queue=w315, element=w312, timeout in ms (-1)=20 ("timeout en ms (-1)"), error in (no error)=w314) -> (queue out=w310:refnum<queue>)  [unwired: 2 out]
                      n114 = Build Array (concatenate)(w312, w311) -> (→"Data":string[][])
                    }
                  }
                }
              }
            }
            frame -1 {
            }
          }
          n115 = Wait Until Next ms Multiple(millisecond multiple=u32 1 ("n millisecondes")) -> ()  [unwired: 1 out]
        }
        "NMEA" <- w244
      }
      frame True {
      }
    }
    n116 = Wait Until Next ms Multiple(millisecond multiple=u32 1 ("n millisecondes")) -> ()  [unwired: 1 out]
  }
  n117 = while {
    stop <- FALSE stop-if-true
    n118 = Random Number (0-1)() -> (number: 0 to 1=w331:dbl)
    n119 = Multiply(x=w331, y=5.0) -> (x*y=w332:dbl)
    n120 = Add(x=w332, y=5.0) -> (x+y=→"Gauge":dbl)
    n121 = Wait (ms)(milliseconds to wait=u32 200) -> ()  [unwired: 1 out]
  }
  n122 = while {
    shift-right: [w333] -> w23
    shift-left: w16 -> [w337]
    tunnel: w18 -> [w336]
    tunnel: [w334] -> w24
    stop <- w339 stop-if-true
    # "Serial Write and Read Loop"
    n123 = case shown="True" "connect" {
      tunnel: [w375 w421] -> w333
      tunnel: w337 -> [w347 w421]
      tunnel: [w373 w420] -> w334
      tunnel: w336 -> [w346 w420]
      frame True {
        (unwired) FALSE
        n124 = VISA Read(VISA resource name=w347, byte count="Read Count", error in (no error)=w346) -> (VISA resource name out=w375:refnum<visa-resource-name>, read buffer=w348:string, error out=w373:errorcluster)  [unwired: 1 out]
        "Response" <- w348
        n125 = Match Pattern(string=w348, regular expression="gyroz:") -> (match substring=w360:string, after substring=w359:string)  [unwired: 1 in, 2 out]
        n126 = Match Pattern(string=w348, regular expression="sicaklik:") -> (match substring=w367:string, after substring=w371:string)  [unwired: 1 in, 2 out]
        n127 = Match Pattern(string=w348, regular expression="basinc:") -> (match substring=w368:string, after substring=w369:string)  [unwired: 1 in, 2 out]
        n128 = Match Pattern(string=w348, regular expression="ivmez:") -> (match substring=w349:string, after substring=w350:string)  [unwired: 1 in, 2 out]
        n129 = Match Pattern(string=w348, regular expression="gyrox:") -> (match substring=w355:string, after substring=w356:string)  [unwired: 1 in, 2 out]
        n130 = Match Pattern(string=w348, regular expression="ivmex:") -> (match substring=w354:string, after substring=w353:string)  [unwired: 1 in, 2 out]
        n131 = Match Pattern(string=w348, regular expression="ry") -> (match substring=w361:string, after substring=w362:string)  [unwired: 1 in, 2 out]
        n132 = Match Pattern(string=w348, regular expression="rx") -> (match substring=w366:string, after substring=w365:string)  [unwired: 1 in, 2 out]
        n133 = case shown="\"gyroz:\"" w360 {
          tunnel: w359 -> [_ w406]
          frame "False", Default {
          }
          frame "gyroz:" {
            n134 = property on="gyro z" class="Str"("Value"=w406) -> ()  [unwired: 2 in, 2 out]
            n135 = Fract/Exp String To Number(use system decimal point (T)=FALSE, string=w406) -> (number=→"Gyro Z":dbl)  [unwired: 2 in, 1 out]
          }
        }
        n136 = case shown="\"sicaklik:\"" w367 {
          tunnel: w371 -> [_ w418]
          frame "False", Default {
          }
          frame "sicaklik:" {
            n137 = property on="Temperature" class="Str"("Value"=w418) -> ()  [unwired: 2 in, 2 out]
            n138 = Fract/Exp String To Number(use system decimal point (T)=FALSE, string=w418) -> (number=→"Temperature" →"Temperature":dbl)  [unwired: 2 in, 1 out]
          }
        }
        n139 = case shown="\"basinc:\"" w368 {
          tunnel: w369 -> [_ w416]
          frame "False", Default {
          }
          frame "basinc:" {
            n140 = property on="BASINÇ" class="Str"("Value"=w416) -> ()  [unwired: 2 in, 2 out]
            n141 = Fract/Exp String To Number(use system decimal point (T)=FALSE, string=w416) -> (number=→"BASINÇ ATM":dbl)  [unwired: 2 in, 1 out]
          }
        }
        n142 = case shown="\"ivmez:\"" w349 {
          tunnel: w350 -> [_ w391]
          frame "False", Default {
          }
          frame "ivmez:" {
            n143 = property on="ivme z" class="Str"("Value"=w391) -> ()  [unwired: 2 in, 2 out]
            n144 = Fract/Exp String To Number(use system decimal point (T)=FALSE, string=w391) -> (number=w389:dbl)  [unwired: 2 in, 1 out]
            n145 = Multiply(x=w389, y=0.001) -> (x*y=→"Gravity":dbl)
          }
        }
        n146 = case shown="\"gyrox:\"" w355 {
          tunnel: w356 -> [_ w404]
          frame "False", Default {
          }
          frame "gyrox:" {
            n147 = Search/Split String(string=w404, search string/char (-)=" ") -> (substring before match=w397:string, match + rest of string=w399:string)  [unwired: 1 in, 1 out]
            n148 = property on="gyro x" class="Str"("Value"=w397) -> ()  [unwired: 2 in, 2 out]
            n149 = Search/Split String(string=w399, search string/char (-)="gyroz:") -> (substring before match=w400:string)  [unwired: 1 in, 2 out]
            n150 = Fract/Exp String To Number(use system decimal point (T)=FALSE, string=w397) -> (number=→"Gyro X":dbl)  [unwired: 2 in, 1 out]
            n151 = Match Pattern(string=w400, regular expression="gyroy:") -> (after substring=w393:string)  [unwired: 1 in, 3 out]
            n152 = property on="gyro y" class="Str"("Value"=w393) -> ()  [unwired: 2 in, 2 out]
            n153 = Fract/Exp String To Number(use system decimal point (T)=FALSE, string=w393) -> (number=→"Gyro Y":dbl)  [unwired: 2 in, 1 out]
          }
        }
        n154 = case shown="\"ivmex:\"" w354 {
          tunnel: w353 -> [_ w387]
          frame "False", Default {
          }
          frame "ivmex:" {
            n155 = Search/Split String(string=w387, search string/char (-)=" ") -> (substring before match=w379:string, match + rest of string=w382:string)  [unwired: 1 in, 1 out]
            n156 = property on="ivme x" class="Str"("Value"=w379) -> ()  [unwired: 2 in, 2 out]
            n157 = Search/Split String(string=w382, search string/char (-)="ivmez:") -> (substring before match=w383:string)  [unwired: 1 in, 2 out]
            n158 = Fract/Exp String To Number(use system decimal point (T)=FALSE, string=w379) -> (number=→"Acceleration X":dbl)  [unwired: 2 in, 1 out]
            n159 = Match Pattern(string=w383, regular expression="ivmey:") -> (after substring=w377:string)  [unwired: 1 in, 3 out]
            n160 = property on="ivme y" class="Str"("Value"=w377) -> ()  [unwired: 2 in, 2 out]
            n161 = Fract/Exp String To Number(use system decimal point (T)=FALSE, string=w377) -> (number=→"Acceleration Y":dbl)  [unwired: 2 in, 1 out]
          }
        }
        n162 = case shown="\"ry\"" w361 {
          tunnel: w362 -> [_ w409]
          tunnel: [_ w408] -> w342
          frame "False", Default {
          }
          frame "ry" {
            n163 = property on="ry" class="Str"("Value"=w409) -> ()  [unwired: 2 in, 2 out]
            n164 = Fract/Exp String To Number(use system decimal point (T)=FALSE, string=w409) -> (number=w408:dbl)  [unwired: 2 in, 1 out]
            "Ry" <- w408
          }
        }
        n165 = case shown="\"rx\"" w366 {
          tunnel: w365 -> [_ w412]
          tunnel: [_ w411] -> w343
          frame "False", Default {
          }
          frame "rx" {
            n166 = property on="rx" class="Str"("Value"=w412) -> ()  [unwired: 2 in, 2 out]
            n167 = Fract/Exp String To Number(use system decimal point (T)=FALSE, string=w412) -> (number=w411:dbl)  [unwired: 2 in, 1 out]
            "Rx" <- w411
          }
        }
        n168 = Build Array(w342) -> (w341:dbl[])
        n169 = Build Array(w343) -> (w345:dbl[])
        n170 = Bundle(w341, w345) -> (→"XY Graph 2":cluster{dbl[], dbl[]})  [unwired: 1 in]
      }
      frame False {
      }
    }
    n171 = Wait Until Next ms Multiple(millisecond multiple=u32 5 ("milliseconds to wait")) -> ()  [unwired: 1 out]
    n172 = Or(x=w334, y="Stop 2") -> (x .or. y?=w339:bool)
  }
  n173 = while {
    shift-right: [w427] -> w64
    shift-left: w60 -> [w433]
    shift-right: [w428] -> w63
    shift-left: w61 -> [w432]
    stop <- w429 stop-if-true
    # "write control"
    n174 = property on="Gyro X" class="Slide (strict)"() -> ("Value"=w424:dbl)  [unwired: 2 in, 2 out]
    n175 = property on="Gyro Y" class="Slide (strict)"() -> ("Value"=w425:dbl)  [unwired: 2 in, 2 out]
    n176 = property on="Gyro Z" class="Slide (strict)"() -> ("Value"=w426:dbl)  [unwired: 2 in, 2 out]
    n177 = Wait (ms)(milliseconds to wait=u32 10) -> ()  [unwired: 1 out]
    n178 = Bundle By Name(cluster="Control 1", "X"=w424, "Y"=w425, "Z"=w426) -> (w422:T11)
    n179 = call "Attitude Control Write.vi"("error in (no error)"=w432, "pitch (x), roll (y), yaw (z)"=w422, "Attitude Control Handle In"=w433) -> ("error out"=w428:errorcluster, "Attitude Control Handle Out"=w427:T16)  [unwired: 7 in]
    n180 = Or(x=w428, y="stop") -> (x .or. y?=w429:bool)
  }
  n181 = while {
    stop <- "pusula stop" stop-if-true
    n182 = Wait Until Next ms Multiple(millisecond multiple=u32 100) -> ()  [unwired: 1 out]
    n183 = Add(x="pusula", y=90.0) -> (x+y=w437:dbl)
    n184 = Compound Arithmetic op=MULTIPLY(w437, 6.283185307179586, invert 360.0 ("value")) -> (w435:dbl)
    n185 = property on="Gauge" class="Knob (strict)"("Scale.SclPosStart"=w435, "Value"="pusula") -> ()  [unwired: 2 in, 2 out]
  }
  n186 = call "Attitude Control Close.vi"("error in (no error)"=w63, "Attitude Control Handle"=w64) -> ("error out"=w65:errorcluster)  [unwired: 9 in]
  n187 = call <vilib>:"Simple Error Handler.vi"("error in (no error)"=w65) -> ()  [unwired: 4 in, 5 out]
  n188 = Release Queue(queue=w46, error in (no error)=w47) -> ()  [unwired: 1 in, 3 out]
  n189 = VISA Close(VISA resource name=w44, error in (no error)=w43) -> (error out=w48:errorcluster)
  n190 = call <vilib>:"Clear Errors.vi"("error in (no error)"=w48) -> ()  [unwired: 5 in, 2 out]
  n191 = VISA Close(VISA resource name=w23, error in (no error)=w24) -> (error out=w25:errorcluster)
  n192 = call <vilib>:"Simple Error Handler.vi"("error in (no error)"=w25) -> ()  [unwired: 1 in, 8 out]
  "Flight Mode" <- "SIMULATING" ("Flight Mode")
